vi "SetWarning.vi"(4 "Append timestamp?":bool caption="Append timestamp? (F)", 6 "Warning label":string="Custom" caption="Warning label (\"Custom\")", 9 "Error in":errorcluster caption="Error in (no error)", 10 "Warning description":string caption="Warning description (\"\")", 11 "Warning code":i32) -> (1 "Error out":errorcluster)   [LabVIEW 2017, in "GPError.lvlib"]
doc: "Sets a warning on <B>Error out</B> if <B>Error in</B> allows it.\n\nIf <B>Error in</B> is 'No error' this VI replaces that with the new warning. If <B>Error in</B> is already a collection of appended errors this VI appends the new warning to that collection.\n\nThe call chain will always be set in <B>Error out</B> source, and description(s) will be appended from one or more of these sources (in the following order):\n\n1) If any built-in or user defined error/warning descriptions exist in LabVIEW's database these will come first.\n\n2) If any custom descriptions are defined for <B>Warning code</B> (with the DefineCustomCode function), these will be appended to the built-in descriptions. If no built-in descriptions exist the custom descriptions are used by themselves.\n\n3) If anything but an empty string is wired to the <B>Warning description</B> input this will be appended to any of the above or used by itself if nothing else is defined. This lets you add a final qualifier or give additional info to the specific warning on top of the pre-defined, and maybe somewhat generic, descriptions (e.g. \"MyWarningHandler: This warning was caused by prolonged loading of X seconds of this specific module\").\n\nThe optional <B>Warning label</B> lets you format the warning description for conformity with built-in LabVIEW warning messages like this: \"<Label>:\\s\\s<Description>\".\n\nThe optional <B>Append timestamp?</B> specifies if the current UTC time and date will be appended to the source string.\n\nThis VI is inlined.\n\nSteen Schmidt\nGPower\n16/7 2013"
uses:
  GPError.lvlib
  Append/AppendSingle.vi
panel:
  # "Copyright © 2013\nSteen Schmidt, GPower\nSee enclosed license file for terms and conditions"
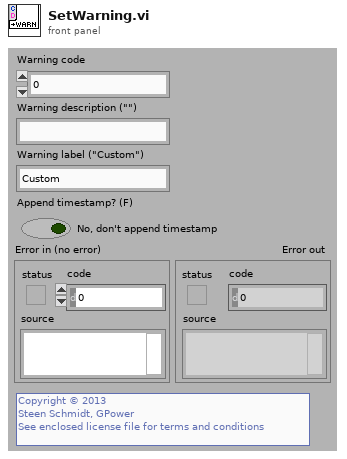
[diagram p1: front panel]
types:
  T1 = typedef "GPError.lvlib/ErrorType.ctl" = enum16{"No Error", "Error", "Warning", "Appended errors", "Appended warnings", "Appended mixed"}
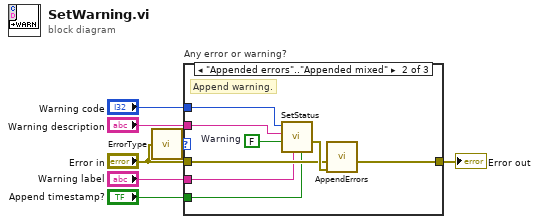
[diagram p0: block diagram]
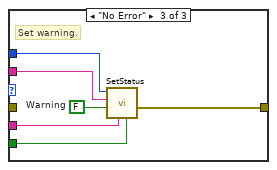
[diagram p3: hidden frame]
diagram:
  n1 = call "ErrorType.vi"("Error in"="Error in") -> ("Error type"=w3:T1)  [unwired: 4 in]
  n2 = case "Any error or warning?" shown="\"Appended errors\"..\"Appended mixed\"" w3 {
    tunnel: [w8 w9 w21] -> w5
    tunnel: "Warning code" -> [_ w11 w19]
    tunnel: "Warning description" -> [_ w12 w20]
    tunnel: "Error in" -> [w8 w14 _]
    tunnel: "Append timestamp?" -> [_ w10 w18]
    tunnel: "Warning label" -> [_ w13 w17]
    frame "Error", "Warning" {
      # "Keep existing error or warning."
    }
    frame "Appended errors".."Appended mixed" {
      w16 = FALSE  # Warning
      # "Append warning."
      n3 = call "SetStatus.vi"("Append timestamp?"=w10, "Label"=w13, "Error?"=w16, "Description"=w12, "Code"=w11) -> ("Error out"=w15:errorcluster)  [unwired: 6 in]
      n4 = call-poly "AppendErrors.vi"("Error to append"=w15, "Error in"=w14) -> ("Appended errors out"=w9:errorcluster)  [unwired: 9 in]
    }
    frame "No Error" {
      w22 = FALSE  # Warning
      # "Set warning."
      n5 = call "SetStatus.vi"("Append timestamp?"=w18, "Label"=w17, "Error?"=w22, "Description"=w20, "Code"=w19) -> ("Error out"=w21:errorcluster)  [unwired: 6 in]
    }
  }
  "Error out" <- w5
